vi "Set String Array Package Attribute Value.vi"(6 "add nonexisting attribute to string (T)":bool=TRUE, 8 "error in (no error)":errorcluster, 9 "package attribute value":string[](array[string]), 10 "package attribute name":string, 11 "package attributes string in":string) -> (0 "error out":errorcluster, 1 "attribute found?":bool, 2 "new attribute added to string?":bool, 3 "package attributes string out":string)   [LabVIEW 2014, in "NIPM_API.lvlib"]
doc: "Sets the value for an attribute in a package attribute string.\n\npackage attributes string in - This is the initial string containing the package attributes. For example, this string could come from reading the contents of an unpacked package's control file.\n\npackage attribute name - This is the name of the attribute whose value you want to change.\n\npackage attribute value - This is the value you want to set the attribute to.\n\nadd nonexisting attribute to string - If this VI does not find the \"package attribute name\" in the \"package attributes string in\" string, this input determines whether this VI will add the \"package attribute name\" and \"package attribute value\" to the \"package attribute string\".\nNote: If this input is TRUE, but the \"package attribute value\" is a default value (\"\"), then this VI will not add a new attribute to the string.\n\nnew attribute added to string? - This output will be TRUE if a new attribute (did not exist in the incoming \"package attributes string in\" string) was added to the package attributes string.\n\nattribute found? - This output will be TRUE if the \"package attribute name\" was found in the incoming \"package attributes string in\" string."
uses:
  NIPM_API.lvlib
  <vilib>/Utility/error.llb/whitespace.ctl
panel:
  # "Refer to the following page for the proper syntax for the package attribute values:\nhttp://www.ni.com/documentation/en/ni-package-manager/latest/manual/control-file-attributes/#GUID-16D97F2A-09D6-4F28-A33C-35D1BBEC07A8"
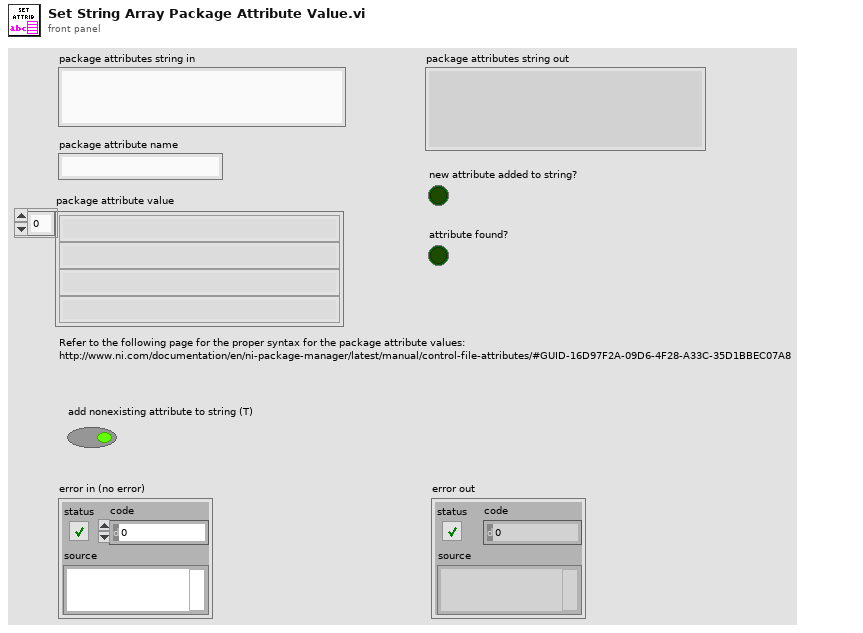
[diagram p1: front panel]
types:
  T1 = typedef "whitespace.ctl" = u16
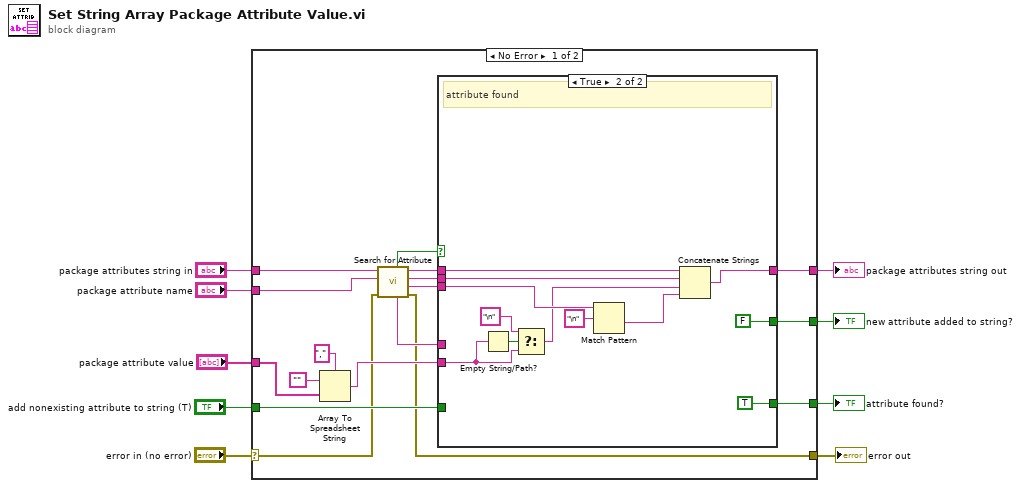
[diagram p0: block diagram]
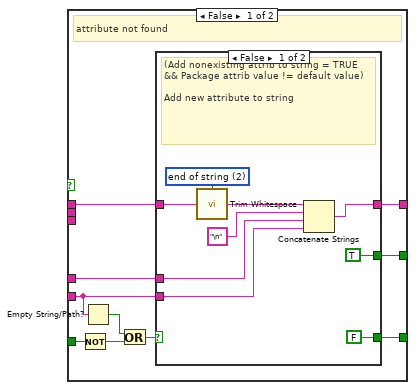
[diagram p2: hidden frame]
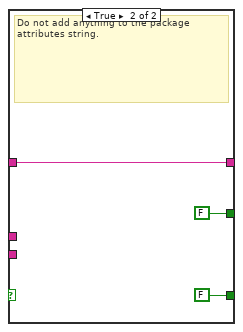
[diagram p3: hidden frame]
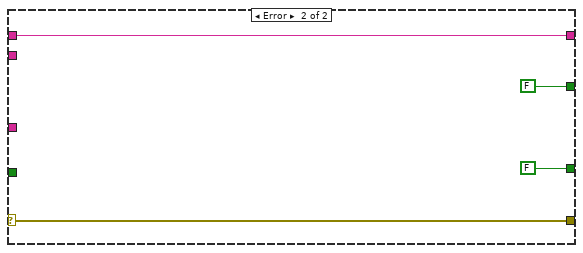
[diagram p4: hidden frame]
diagram:
  n1 = case shown="No Error" "error in (no error)" {
    selector: "error in (no error)" -> [w11 w64]
    tunnel: [w26 w61] -> w9
    tunnel: "package attribute name" -> [w17 _]
    tunnel: "package attributes string in" -> [w18 w61]
    tunnel: [w10 w64] -> w5
    tunnel: "package attribute value" -> [w20 _]
    tunnel: [w25 FALSE] -> w4
    tunnel: "add nonexisting attribute to string (T)" -> [w24 _]
    tunnel: [w23 FALSE] -> w2
    frame No Error {
      n2 = Array To Spreadsheet String(delimiter (Tab)=",", array=w20, 3:"") -> (spreadsheet string=w19:string)
      n3 = call "Search for Attribute.vi"("error in (no error)"=w11, "package attribute name"=w17, "package attributes CLI string in"=w18) -> ("error out"=w10:errorcluster, "string after attribute"=w14:string, "string matching attribute"=w15:string, "string before attribute"=w16:string, "package attribute string"=w12:string, "attribute found?"=w13:bool)  [unwired: 3 in]
      n4 = case shown="True" w13 {
        tunnel: w16 -> [w36 w60]
        tunnel: w15 -> [_ w59]
        tunnel: w19 -> [w27 w50]
        tunnel: w14 -> [_ w58]
        tunnel: [w34 w56] -> w26
        tunnel: [w35 FALSE] -> w25
        tunnel: w12 -> [w33 _]
        tunnel: w24 -> [w32 _]
        tunnel: [w31 TRUE] -> w23
        frame False {
          # "attribute not found"
          n5 = Not(x=w32) -> (.not. x?=w30:bool)
          n6 = Empty String/Path?(string/path=w27) -> (empty?=w28:bool)
          n7 = Or(x=w28, y=w30) -> (x .or. y?=w29:bool)
          n8 = case shown="False" w29 {
            tunnel: w36 -> [w45 w48]
            tunnel: [TRUE FALSE] -> w35
            tunnel: [w43 w48] -> w34
            tunnel: w33 -> [w42 _]
            tunnel: w27 -> [w41 _]
            tunnel: [FALSE FALSE] -> w31
            frame False {
              w39 = T1 2 items=["both", "start of string", "end of string"] ("location (both)")
              # "(Add nonexisting attrib to string = TRUE && Package attrib value != default value)\n\nAdd new attribute to string"
              n9 = call <vilib>:"Trim Whitespace.vi"("string"=w45, "location (both)"=w39) -> ("trimmed string"=w40:string)
              n10 = Concatenate Strings(w40, "\n", w42, w41) -> (w43:string)
            }
            frame True {
              # "Do not add anything to the package attributes string."
            }
          }
        }
        frame True {
          # "attribute found"
          n11 = Empty String/Path?(string/path=w50) -> (empty?=w52:bool)
          n12 = Select(t="\n" ("regular expression"), s=w52, f=w50) -> (s? t:f=w49:string)
          n13 = Match Pattern(string=w58, regular expression="\n") -> (after substring=w53:string)  [unwired: 1 in, 3 out]
          n14 = Concatenate Strings(w60, w59, w49, w53) -> (w56:string)
        }
      }
    }
    frame Error {
    }
  }
  "package attributes string out" <- w9
  "error out" <- w5
  "new attribute added to string?" <- w4
  "attribute found?" <- w2
